vi "Initialize AO Channels.vi"(8 "error in (no error)":errorcluster, 11 "Instrument.Lockin in":refnum<class "Instrument.Lockin.lvclass">) -> (0 "error out":errorcluster, 3 "Instrument.Lockin out":refnum<class "Instrument.Lockin.lvclass">)   [LabVIEW 2016, in "LockinDAQ.lvclass"]
uses:
  LockinDAQ.lvclass
  Typedefs/Function-enum.ctl
  Instrument.Lockin/Instrument.Lockin.lvclass
  C:/Program Files (x86)/National Instruments/LabVIEW 2016/user.lib/LevyLab/Levylab Instruments/SMOs/Instrument/Instrument.lvclass
  C:/Program Files (x86)/National Instruments/LabVIEW 2016/user.lib/LevyLab/Levylab Instruments/SMOs/LevyLab/LevyLab.lvclass
  C:/Program Files (x86)/National Instruments/LabVIEW 2016/vi.lib/JKI/JKI SMO/SMO/SMO.lvclass
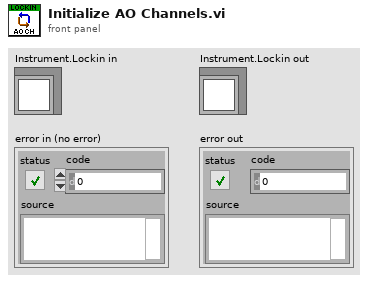
[diagram p1: front panel]
types:
  T1 = typedef "LockinDAQ.lvclass/Function-enum.ctl" = enum16{"Sine", "Triangle", "Square", "Sawtooth"}
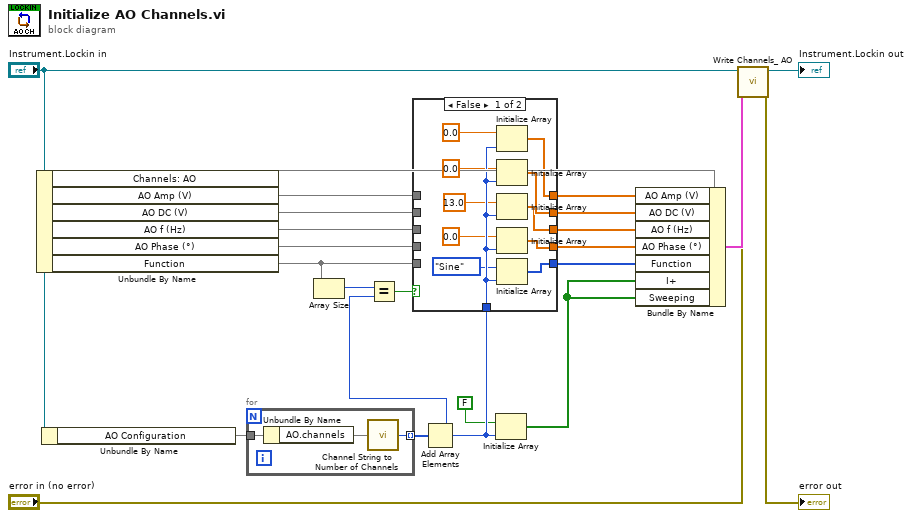
[diagram p0: block diagram]
diagram:
  n1 = Unbundle By Name("Instrument.Lockin in") -> ("Channels: AO"=w21, "AO Amp (V)"=w16, "AO DC (V)"=w17, "AO f (Hz)"=w18, "AO Phase (°)"=w19, "Function"=w20)
  n2 = Unbundle By Name("Instrument.Lockin in") -> ("AO Configuration"=w15)
  n3 = for {
    tunnel: w15 -> [w26]
    tunnel: [w24] -> w4 mode=indexing
    n4 = Unbundle By Name(w26) -> ("AO.channels"=w25)
    n5 = call "Channel String to Number of Channels.vi"("Channels String"=w25) -> ("# channels"=w24:i32)  [unwired: 4 in]
  }
  n6 = Array Size(array=w20) -> (size(s)=w6:i32)
  n7 = Add Array Elements(numeric array=w4) -> (sum=w14:i32)
  n8 = Equal?(x=w6, y=w14) -> (x = y?=w8:bool)
  n9 = case shown="False" w8 {
    tunnel: [w35 w42] -> w9
    tunnel: w20 -> [_ w42]
    tunnel: [w34 w38] -> w10
    tunnel: [w32 w41] -> w11
    tunnel: w18 -> [_ w41]
    tunnel: [w33 w40] -> w12
    tunnel: w17 -> [_ w40]
    tunnel: [w36 w39] -> w13
    tunnel: w16 -> [_ w39]
    tunnel: w14 -> [w37 _]
    tunnel: w19 -> [_ w38]
    frame False {
      n10 = Initialize Array(0.0, w37) -> (w36:dbl[])
      n11 = Initialize Array(0.0, w37) -> (w33:dbl[])
      n12 = Initialize Array(13.0, w37) -> (w32:dbl[])
      n13 = Initialize Array(0.0, w37) -> (w34:dbl[])
      n14 = Initialize Array(Function-enum."Sine" ("Signal Type"), w37) -> (w35:T1[])
    }
    frame True {
    }
  }
  n15 = Initialize Array(FALSE, w14) -> (w7:bool[])
  n16 = Bundle By Name(cluster=w21, "AO Amp (V)"=w13, "AO DC (V)"=w12, "AO f (Hz)"=w11, "AO Phase (°)"=w10, "Function"=w9, "I+"=w7, "Sweeping"=w7) -> (w22:cluster{})
  n17 = call "Write Channels_ AO.vi"("error in (no error)"="error in (no error)", "Channels: AO"=w22, "Instrument.Lockin in"="Instrument.Lockin in") -> ("error out"=→"error out":errorcluster, "Instrument.Lockin out"=→"Instrument.Lockin out":refnum<class "Instrument.Lockin.lvclass">)  [unwired: 7 in]
